vi "Test Compare Array of Strings.vi"(8 "error in (no error)":errorcluster, 11 "Test Case In":refnum<class "Comparator Message Test.lvclass">) -> (0 "error out":errorcluster, 3 "Test Case Out":refnum<class "Comparator Message Test.lvclass">)   [LabVIEW 2020, in "Comparator Message Test.lvclass"]
uses:
  Comparator Message Test.lvclass
  source/Comparators/Identical Arguments Comparator/Identical Inputs Comparator.lvclass
  C:/git/astemes-lmock/source/Core/Comparator/Comparator.lvclass
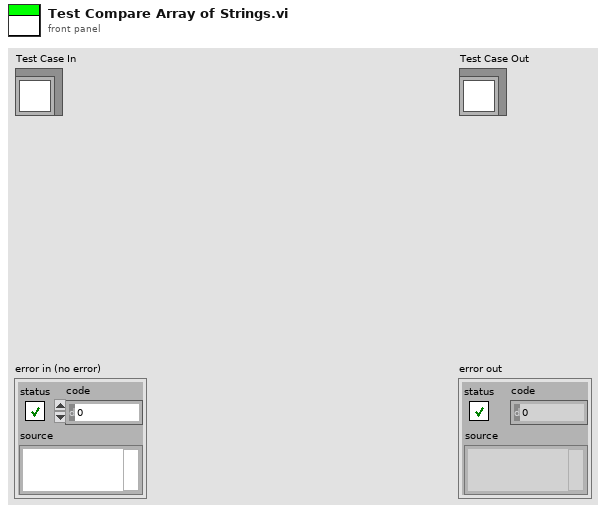
[diagram p1: front panel]
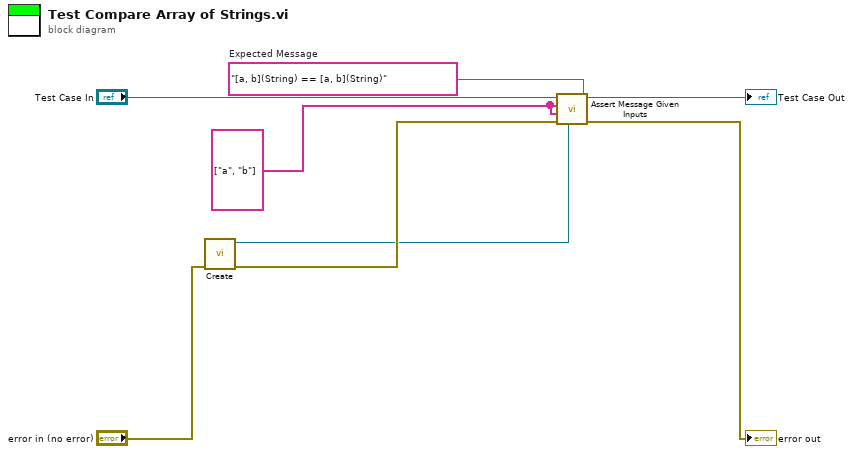
[diagram p0: block diagram]
diagram:
  w3 = "[a, b](String) == [a, b](String)"  # Expected Message
  w1 = string[] ["a", "b"]
  n1 = call "Create.vi"("error in (no error)"="error in (no error)") -> ("error out"=w5:errorcluster, "Identical Inputs Comparator"=w2:refnum<class "Identical Inputs Comparator.lvclass">)  [unwired: 9 in]
  n2 = call "Assert Message Given Inputs.vi"("Identical Inputs Comparator"=w2, "Expected Message"=w3, "error in (no error)"=w5, "Call 2"=w1, "Call 1"=w1, "Comparator Message Test in"="Test Case In") -> ("error out"=→"error out":errorcluster, "Comparator Message Test out"=→"Test Case Out":refnum<class "Comparator Message Test.lvclass">)  [unwired: 4 in]
